vi "practice 1.vi"() -> ()   [LabVIEW 2018]
panel:
  in  "数値 7":dbl
  out "文字列 2":string
  in  "数値 6":dbl
  out "数値 5":dbl
  out "数値 4":dbl
  out "数値 3":dbl
  out "波形チャート":dbl(graph)
  out "ブール 2":bool
  out "ゲージ":dbl(knob) scale=0.0..1.0
  in  "ダイアル":dbl(knob) scale=0.0..1.0
  in  "停止":bool
  out "繰り返し回数":dbl
  out "さいころ":i8
  in  "スライド":dbl(slide) scale=0.0..10.0
  out "数値":dbl
  in  "数値 2":dbl
  out "文字列":string
  in  "タイム":string
  out "ブール":bool
  in  "?":bool
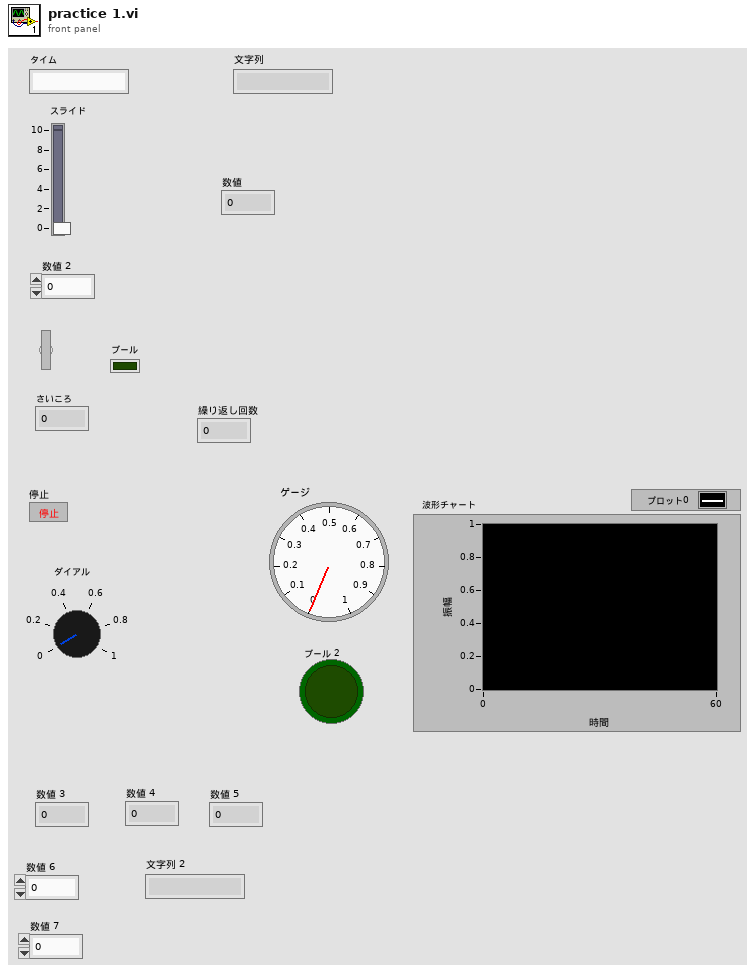
[diagram p1: front panel]
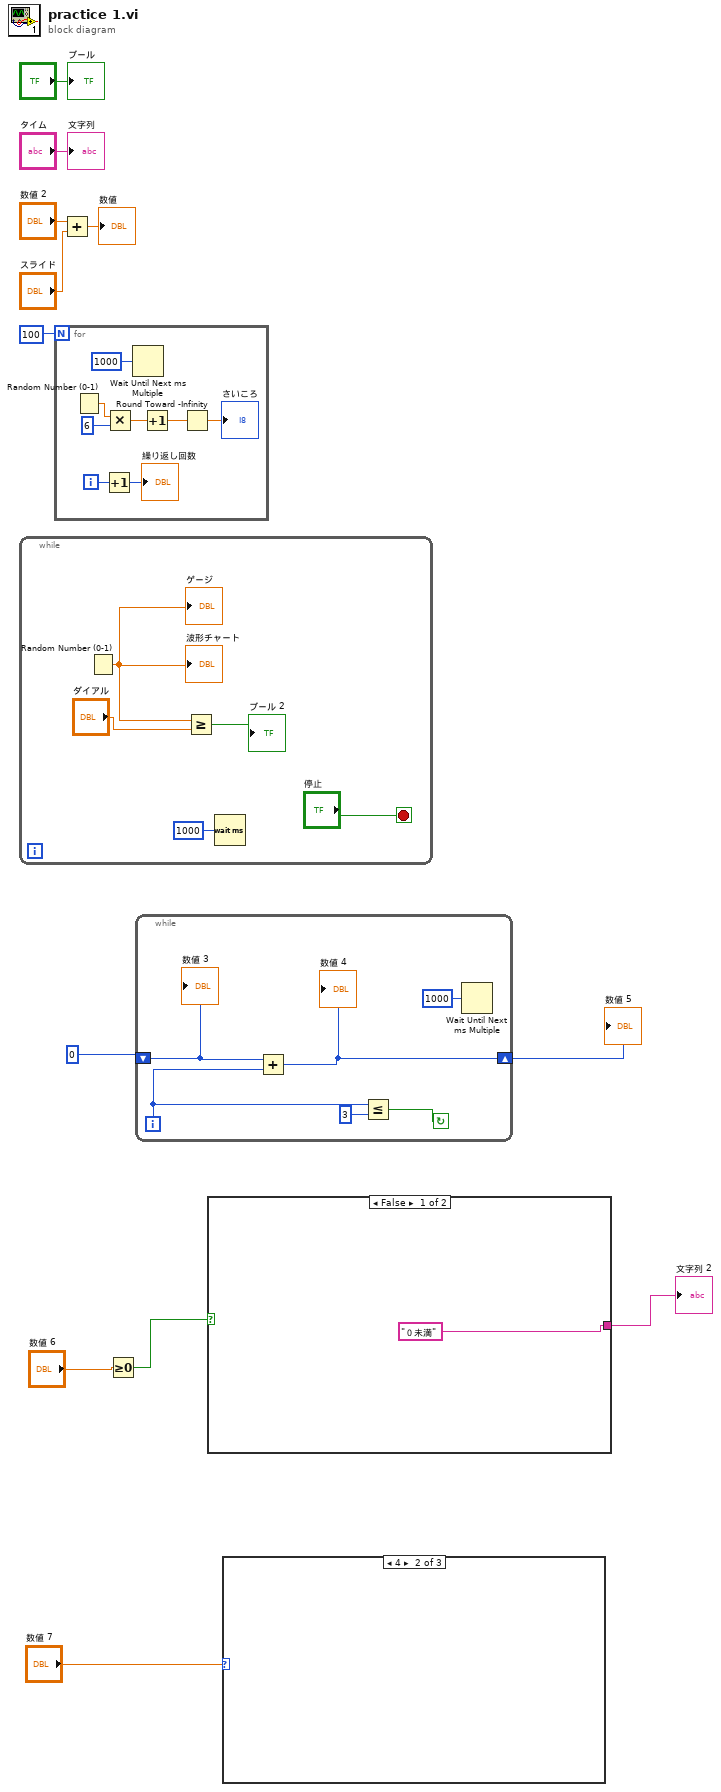
[diagram p0: block diagram]
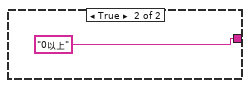
[diagram p4: hidden frame]
diagram:
  n1 = while {
    stop <- "停止" stop-if-true
    n2 = Random Number (0-1)() -> (number: 0 to 1=w15:dbl)
    "ゲージ" <- w15
    "波形チャート" <- w15
    n3 = Greater Or Equal?(x=w15, y="ダイアル") -> (x >= y?=→"ブール 2":bool)
    n4 = Wait (ms) ("待機 (ms)")(milliseconds to wait=u32 1000 ("ミリ秒待機時間")) -> ()  [unwired: 1 out]
  }
  n5 = for {
    N: 100 -> [_]
    i -> [w20]
    n6 = Random Number (0-1)() -> (number: 0 to 1=w25:dbl)
    n7 = Increment(x=w20) -> (x+1=→"繰り返し回数":i32)
    n8 = Multiply(x=w25, y=6) -> (x*y=w23:dbl)
    n9 = Wait Until Next ms Multiple(millisecond multiple=1000) -> ()  [unwired: 1 out]
    n10 = Increment(x=w23) -> (x+1=w22:dbl)
    n11 = Round Toward -Infinity(1:w22) -> (0:→"さいころ":dbl)
  }
  n12 = Add(x="数値 2", y="スライド") -> (x+y=→"数値":dbl)
  n13 = Greater Or Equal To 0?(x="数値 6") -> (x >= 0?=w3:bool)
  n14 = while {
    shift-right: [w27] -> w5
    shift-left: 0 -> [w31]
    i -> [w29]
    stop <- w30 continue-if-true
    n15 = Add(x=w31, y=w29) -> (x+y=w27:i32)
    "数値 4" <- w27
    n16 = Less Or Equal?(x=w29, y=3) -> (x <= y?=w30:bool)
    n17 = Wait Until Next ms Multiple(millisecond multiple=u32 1000 ("ミリ秒倍数")) -> ()  [unwired: 1 out]
    "数値 3" <- w31
  }
  "数値 5" <- w5
  n18 = case shown="FALSE" w3 {
    tunnel: ["０未満" "0以上"] -> w2
    frame False {
    }
    frame True {
    }
  }
  "文字列 2" <- w2
  n19 = case shown="4" "数値 7" {
    frame 1..3 {
    }
    frame 4 {
    }
    frame 1 {
    }
  }
  "ブール" <- "?"
  "文字列" <- "タイム"
